vi "Front.vi"() -> ()   [LabVIEW 2021]
uses:
  TypeDef/Configure I2C Bus timing.ctl
  TypeDef/Pin Levels Configuration.ctl
  Demo_client/RPC Messages/Communication_ActionReply.ctl
  Demo_client/RPC Messages/Communication_ActionRequest.ctl
  Demo_client/Demo_client.lvlib
panel:
  out "I2C Pin Levels Response":T1
  out "Configure I2C Bus timing Response":T1
  in  "I2C Pin Levels":T2={"SCL VIH (V)"=0.0, "SCL VIL (V)"=0.0, "SCL Termination Mode"="Internal", "SCL Load Current (A)"=0.0015, "SDA VIH (V)"=0.0, "SDA VIL (V)"=0.0, "SDA Termination Mode"="Internal", "SDA Load Current (A)"=0.0015, "ModSeIL Termination Mode"="Internal", "ModSeIL VIL (V)"=0.0, "ModSeIL VIH (V)"=1.8} {"ModSeIL VIH (V)" min=-2.0 max=6.0 step=0.1 format="%#_2g"; "ModSeIL VIL (V)" min=-2.0 max=6.0 step=0.1 format="%#_2g"; "SDA Load Current (A)" min=0.0015 max=0.024 step=0.001 format="%#_2p"; "SDA VIH (V)" min=-2.0 max=6.0 step=0.1 format="%#_3g"; "SDA VIL (V)" min=-2.0 max=6.0 step=0.1 format="%#_3g"; "SCL Load Current (A)" min=0.0015 max=0.024 step=0.001 format="%#_2p"; "SCL VIH (V)" min=-2.0 max=6.0 step=0.1 format="%#_3g"; "SCL VIL (V)" min=-2.0 max=6.0 step=0.1 format="%#_3g"}
  in  "Configure I2C Bus timing":T3={"Frequency(Hz)"=10000.0, "T_HIGH(ns)"=0.0, "T_LOW(ns)"=0.0, "T_SU_STO(ns)"=0.0, "T_SU_STA(ns)"=0.0, "T_SU_DAT(ns)"=0.0, "T_BUF(ns)"=0.0, "T_HD_STA(ns)"=0.0, "T_HD_DAT(ns)"=0.0, "T.SU_ModSeIL(ns)"=40000.0, "T.HD_ModSeIL(ns)"=40000.0} {"T.HD_ModSeIL(ns)" min=40000.0 step=40000.0 format="%#_6p"; "T.SU_ModSeIL(ns)" min=40000.0 step=40000.0 format="%#_6p"; "Frequency(Hz)" min=10000.0 max=25000000.0 step=100.0 format="%#_6p"; "T_HD_DAT(ns)" step=1.0 format="%#_5g"; "T_SU_STA(ns)" min=0.0 step=1.0 format="%#_5g"; "T_HD_STA(ns)" min=0.0 step=1.0 format="%#_5g"; "T_SU_STO(ns)" min=0.0 step=1.0 format="%#_5g"; "T_BUF(ns)" min=0.0 step=1.0 format="%#_5g"; "T_HIGH(ns)" min=0.0 step=1.0 format="%#_5g"; "T_LOW(ns)" min=0.0 step=1.0 format="%#_5g"; "T_SU_DAT(ns)" step=1.0 format="%#_5g"}
  # "Pin Levels Configuration"
  # "SCL"
  # "SDA"
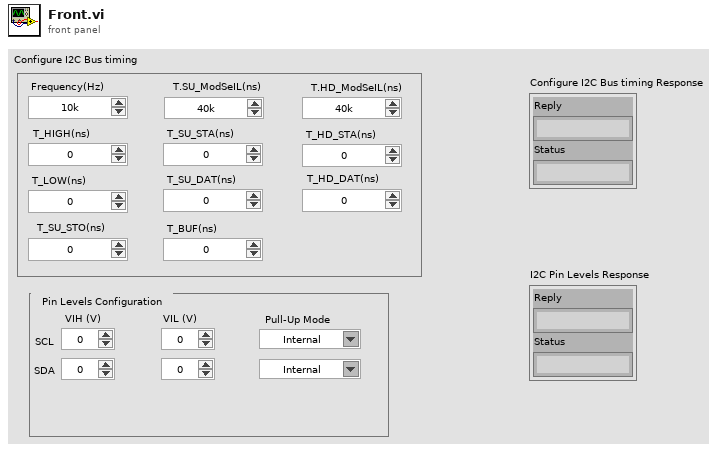
[diagram p1: front panel]
types:
  T1 = typedef "Demo_client.lvlib/Communication_ActionReply.ctl" = cluster{"Reply":string, "Status":string}
  T2 = typedef "Pin Levels Configuration.ctl" = cluster{"SCL VIH (V)":dbl, "SCL VIL (V)":dbl, "SCL Termination Mode":string, "SCL Load Current (A)":dbl, "SDA VIH (V)":dbl, "SDA VIL (V)":dbl, "SDA Termination Mode":string, "SDA Load Current (A)":dbl, "ModSeIL Termination Mode":string, "ModSeIL VIL (V)":dbl, "ModSeIL VIH (V)":dbl}
  T3 = typedef "Configure I2C Bus timing.ctl" = cluster{"Frequency(Hz)":dbl, "T_HIGH(ns)":dbl, "T_LOW(ns)":dbl, "T_SU_STO(ns)":dbl, "T_SU_STA(ns)":dbl, "T_SU_DAT(ns)":dbl, "T_BUF(ns)":dbl, "T_HD_STA(ns)":dbl, "T_HD_DAT(ns)":dbl, "T.SU_ModSeIL(ns)":dbl, "T.HD_ModSeIL(ns)":dbl}
  T4 = typedef "grpc-lvsupport-release.lvlib/grpcId.ctl" = u64
  T5 = typedef "Demo_client.lvlib/Communication_ActionRequest.ctl" = cluster{"Request":string, "Data":string}
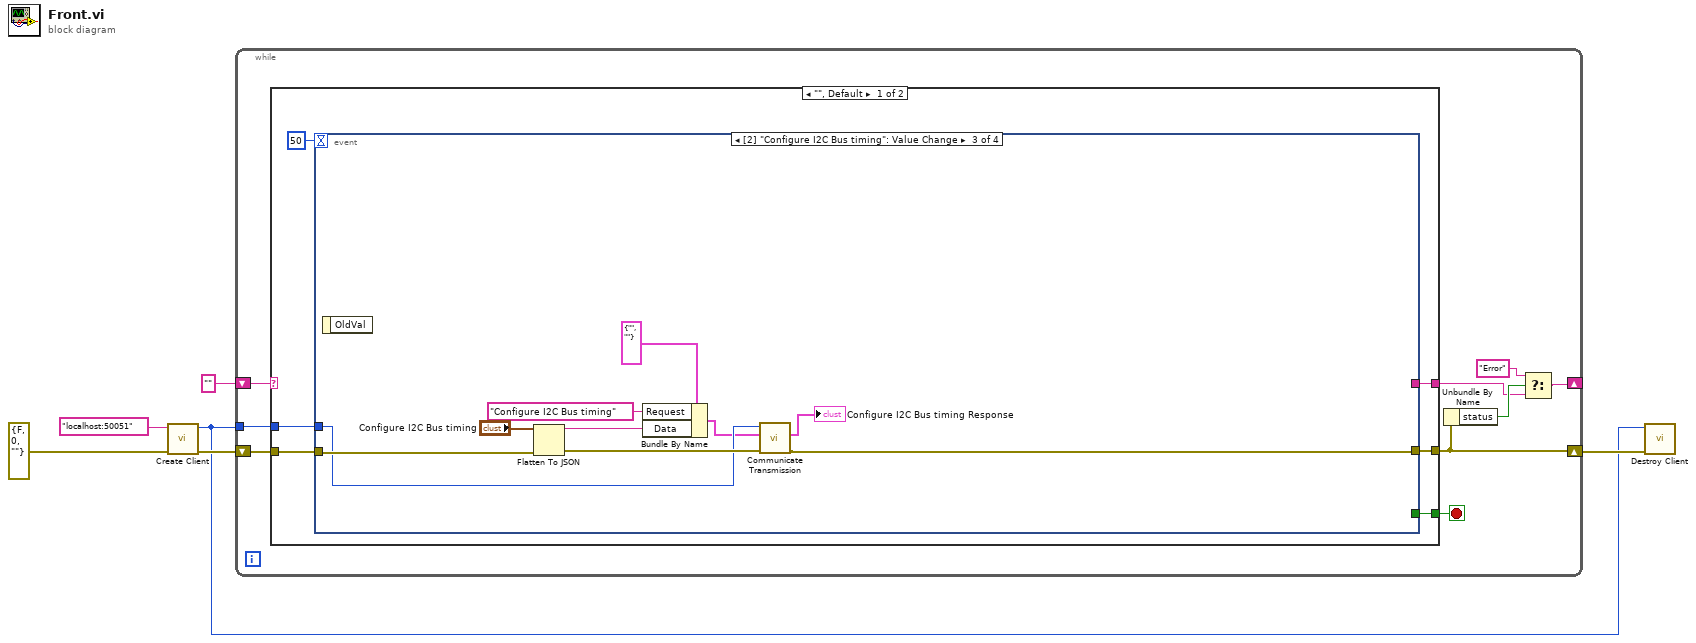
[diagram p0: block diagram]
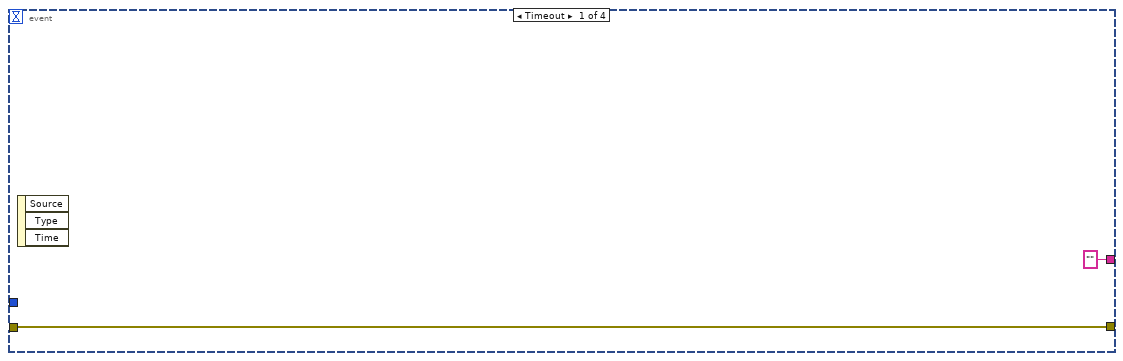
[diagram p2: hidden frame]
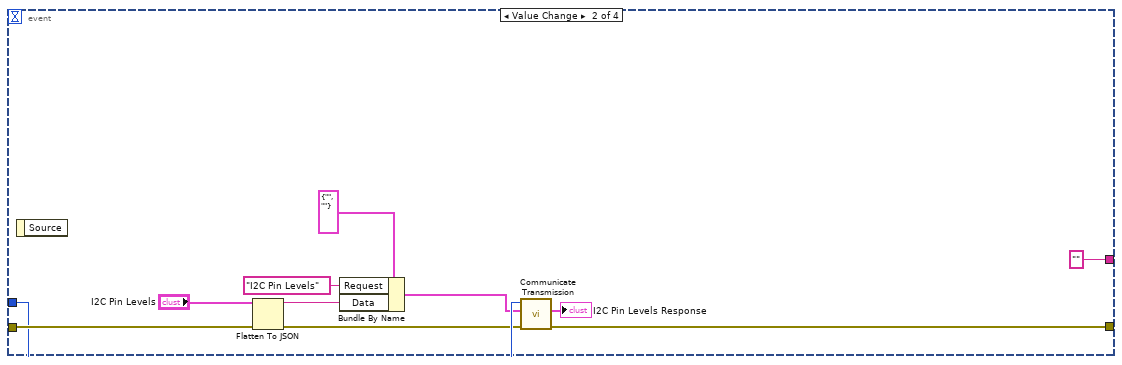
[diagram p3: hidden frame]
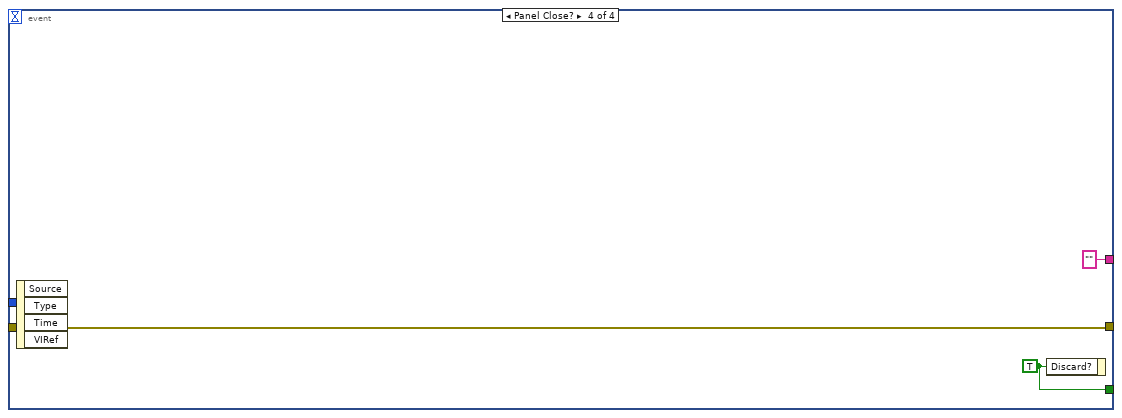
[diagram p4: hidden frame]
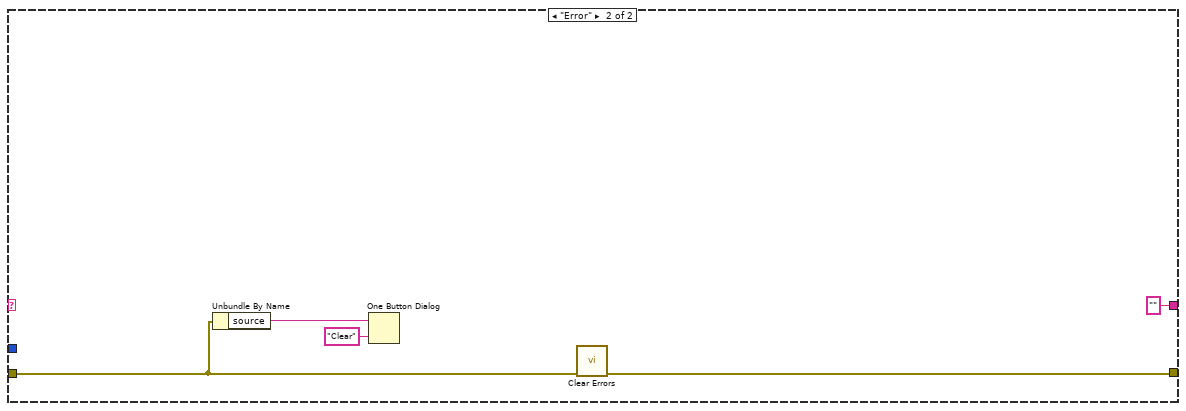
[diagram p5: hidden frame]
diagram:
  n1 = call "Create Client.vi"("error in"=errorcluster {"status"=FALSE, "code"=0, "source"=""} ("error in (no error)"), "address"="localhost:50051") -> ("error out"=w5:errorcluster, "gRPC ID Out"=w1:T4)  [unwired: 8 in]
  n2 = while {
    shift-right: [w11] -> w2
    shift-left: w5 -> [w14]
    tunnel: w1 -> [w13]
    shift-right: [w9] -> _
    shift-left: "" -> [w15]
    stop <- w12 stop-if-true
    n3 = case shown="\"\", Default" w15 {
      tunnel: w14 -> [w21 w51]
      tunnel: [w20 w52] -> w11
      tunnel: w13 -> [w19 _]
      tunnel: [w18 ""] -> w8
      tunnel: [w17 _] -> w12
      frame "", Default {
        n4 = event shown="[2] \"Configure I2C Bus timing\": Value Change" {
          selector: _ -> [_ _ _ _]
          dyn-events: _ -> [_ _ _ _]
          timeout: 50 -> [_ _ _ _]
          tunnel: w21 -> [w23 w32 w43 w47]
          tunnel: [w23 w33 w40 w47] -> w20
          tunnel: w19 -> [_ w31 w38 _]
          tunnel: ["" "" _ ""] -> w18
          tunnel: [_ _ _ w45] -> w17
          event Timeout {
            n5 = event-data() -> ()  [unwired: 1 in, 3 out]
          }
          event Value Change {
            n6 = event-data() -> ()  [unwired: 1 in, 1 out]
            n7 = Flatten To JSON(anything="I2C Pin Levels", error in (no error)=w32) -> (JSON string=w27:string, 11:w30:errorcluster)  [unwired: 1 in]
            n8 = Bundle By Name(cluster=T5 {"Request"="", "Data"=""} ("Request Data"), "Request"="I2C Pin Levels", "Data"=w27) -> (w25:T5)
            n9 = call "Communicate Transmission.vi"("error in"=w30, "Request Data"=w25, "gRPC ID"=w31) -> ("error out"=w33:errorcluster, "Response Data"=→"I2C Pin Levels Response":T1)  [unwired: 6 in, 1 out]
          }
          event Value Change {
            n10 = event-data() -> ()  [unwired: 1 in, 1 out]
            n11 = Flatten To JSON(anything="Configure I2C Bus timing", error in (no error)=w43) -> (JSON string=w42:string, 11:w39:errorcluster)  [unwired: 1 in]
            n12 = Bundle By Name(cluster=T5 {"Request"="", "Data"=""} ("Request Data"), "Request"="Configure I2C Bus timing", "Data"=w42) -> (w37:T5)
            n13 = call "Communicate Transmission.vi"("error in"=w39, "Request Data"=w37, "gRPC ID"=w38) -> ("error out"=w40:errorcluster, "Response Data"=→"Configure I2C Bus timing Response":T1)  [unwired: 6 in, 1 out]
          }
          event Panel Close? {
            w45 = TRUE ("Discard?")
            n14 = event-data() -> ()  [unwired: 1 in, 4 out]
            n15 = event-data("Discard?"=w45) -> ()  [unwired: 1 in, 1 out]
          }
        }
      }
      frame "Error" {
        n16 = Unbundle By Name(w51) -> ("source"=w49:string)
        n17 = One Button Dialog(message=w49, button name ("OK")="Clear") -> ()  [unwired: 1 out]
        n18 = call <vilib>:"Clear Errors.vi"("error in (no error)"=w51) -> ("error out"=w52:errorcluster)  [unwired: 5 in, 1 out]
      }
    }
    n19 = Unbundle By Name(w11) -> ("status"=w10:bool)
    n20 = Select(t="Error", s=w10, f=w8) -> (s? t:f=w9:string)
  }
  n21 = call "Destroy Client.vi"("error in"=w2, "gRPC ID"=w1) -> ()  [unwired: 9 in, 1 out]
